vi "MM6.get i attribute.vi"(0 "i ref in":refnum<vi>, 5 "error in (no error)":errorcluster) -> (14 "i ref out":refnum<vi>, 16 "i attribute":T1={"ConfigData"={"GenConfig"={"Mode"=0, "Logs"=[]}, "Configs"=[]}, "UsedObjs"=[], "ActScanStep"=[], "AbortRequest"=FALSE, "StopRequest"=FALSE, "# cycles"=0, "Connected"=FALSE, "MMStatus"=enum."config", "# data"=0, "DIMServices"={"MM6StatusString"="", "MM6StatusID"=-1, "discArchiver"="", "discArchiverID"=-1, "eventBuilder"="", "eventBuilderID"=-1, "GUIIDString"="", "GUIIDStringID"=-1}, "dataFile"="", "ExtraDataSets"=[], "PGRunning"=0} {"ConfigData"."Configs"."CleanDev"."CleanData"."Time" format="%.3f"; "ConfigData"."Configs"."CleanDev"."CleanData"."Minus" format="%.2f"; "ConfigData"."Configs"."CleanDev"."CleanData"."Plus" format="%.2f"; "ConfigData"."Configs"."CleanDev"."CleanData"."Center" format="%.4f"; "ConfigData"."Configs"."CleanDev"."CleanData"."Amp" format="%.2f"; "ConfigData"."Configs"."Delays"."Delay" format="%.2f"; "ConfigData"."Configs"."Specials"."Data" format="%.2f"; "ConfigData"."Configs"."FreqDevs"."Time" format="%.3f"; "ConfigData"."Configs"."FreqDevs"."CenterFreq" format="%.4f"; "ConfigData"."Configs"."FreqDevs"."Amp" format="%.2f"; "ConfigData"."Configs"."Scans"."Values" format="%.2f"}, 19 "error out":errorcluster)   [LabVIEW 2014, in "MM6.lvlib"]
doc: "Gets the i attribute data of an object.\n\nLicense Agreement for this software:\n\nCopyright (C)\nGesellschaft für Schwerionenforschung, GSI\nPlanckstr. 1\n64291 Darmstadt\nGermany\n\nContact: D.Beck@gsi.de \n\nThis program is free software; you can redistribute it and/or modify it under the terms of the GNU General Public License as published by the Free Software Foundation; either version 2 of the license, or (at your option) any later version.\n\nThis program is distributed in the hope that it will be useful, but WITHOUT ANY WARRANTY; without even the implied warranty of MERCHANTABILITY or FITNESS FOR A PARTICULAR PURPOSE. See the GNU General License for more details (http://www.gnu.org).\n\nGesellschaft für Schwerionenforschung, GSI\nPlanckstr. 1, 64291 Darmstadt, Germany\nFor all questions and ideas contact: M.Richter@gsi.de, H.Brand@gsi.de or D.Beck@gsi.de.\nLast update: 17-JUN-2004"
uses:
  MM6.lvlib
  MM6.i attribute.ctl
  LEBITDefs/LEBITDefs.ConfigData.ctl
  LEBITDefs/LEBITDefs.GenConfig.ctl
  LEBITDefs/LEBITDefs.Log.ctl
  LEBITDefs/LEBITDefs.OneConfig.ctl
  LEBITDefs/LEBITDefs.MCA.ctl
  LEBITDefs/LEBITDefs.Timing.ctl
  LEBITDefs/LEBITDefs.Timetable.ctl
  LEBITDefs/LEBITDefs.Memory.ctl
  LEBITDefs/LEBITDefs.ScanDev.ctl
  LEBITDefs/LEBITDefs.FreqDev.ctl
  LEBITDefs/LEBITDefs.CleanDev.ctl
  LEBITDefs/LEBITDefs.CleanDataType.ctl
  LEBITDefs/LEBITDefs.Special.ctl
  LEBITDefs/LEBITDefs.Delay.ctl
  LEBITDefs/LEBITDefs.DAC.ctl
  MM6.status.ctl
  LEBITDefs/LEBITDefs.ExtraData.ctl
  CS_DigitalIO/PPG_ABC/PPG_ABC.PG_Running.ctl
  LEBITDefs/LEBITDefs.lvlib
  CS_DigitalIO/PPG_ABC/PPG_ABC.lvlib
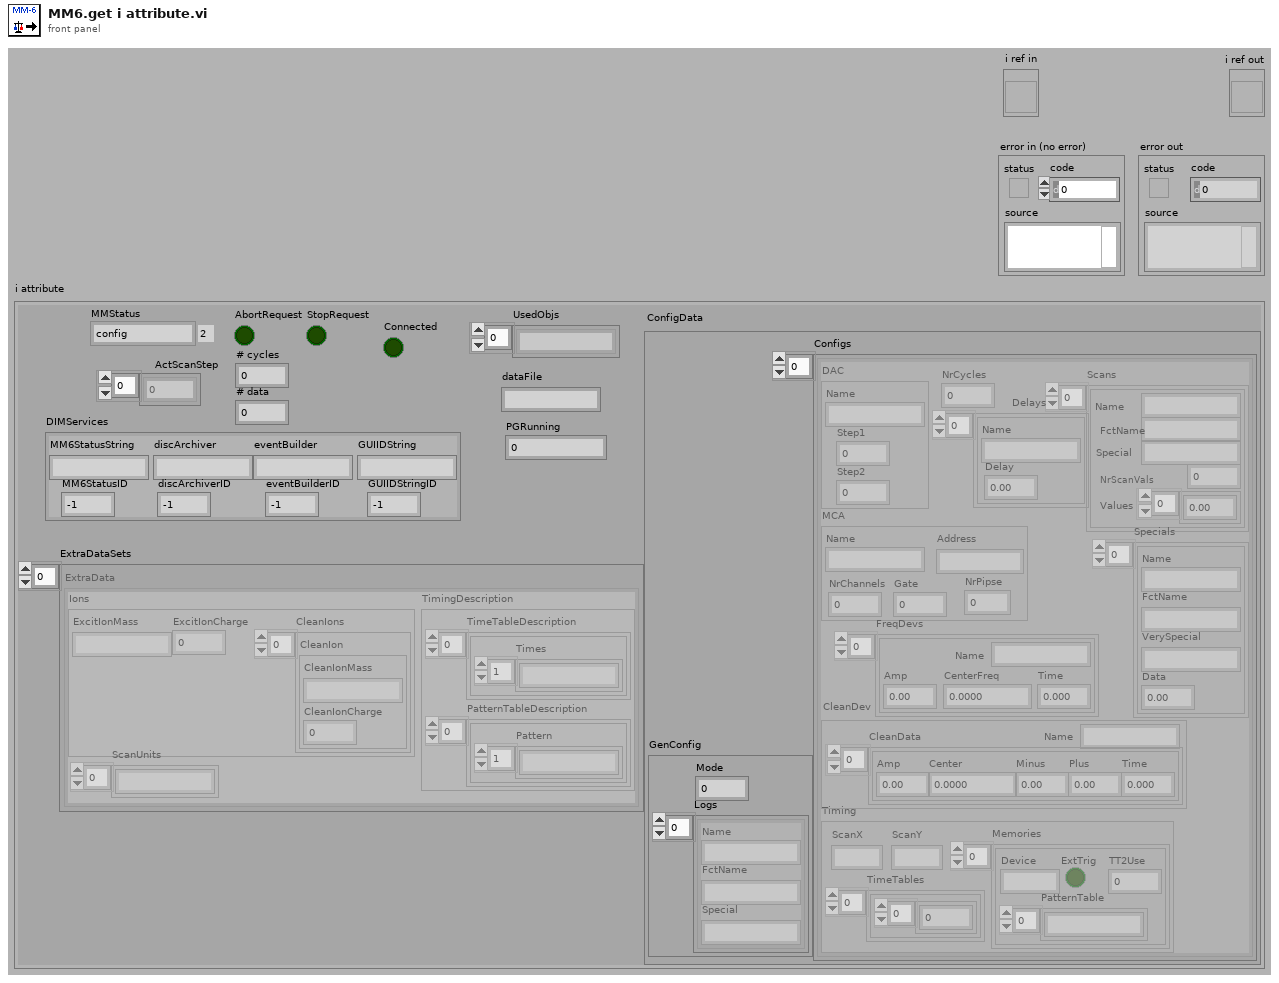
[diagram p1: front panel]
types:
  T1 = typedef "MM6.lvlib/MM6.i attribute.ctl" = cluster{"ConfigData":T2, "UsedObjs":string[], "ActScanStep":i32[], "AbortRequest":bool, "StopRequest":bool, "# cycles":i32, "Connected":bool, "MMStatus":T17, "# data":i32, "DIMServices":cluster{"MM6StatusString":string, "MM6StatusID":i32, "discArchiver":string, "discArchiverID":i32, "eventBuilder":string, "eventBuilderID":i32, "GUIIDString":string, "GUIIDStringID":i32}, "dataFile":string, "ExtraDataSets":T18, "PGRunning":T19}
  T2 = typedef "LEBITDefs.lvlib/LEBITDefs.ConfigData.ctl" = cluster{"GenConfig":T3, "Configs":T5[]}
  T3 = typedef "LEBITDefs.lvlib/LEBITDefs.GenConfig.ctl" = cluster{"Mode":i32, "Logs":T4[]}
  T4 = typedef "LEBITDefs.lvlib/LEBITDefs.Log.ctl" = cluster{"Name":string, "FctName":string, "Special":string}
  T5 = typedef "LEBITDefs.lvlib/LEBITDefs.OneConfig.ctl" = cluster{"MCA":T6, "Timing":T7, "Scans":T10[], "FreqDevs":T11[], "CleanDev":T12, "NrCycles":i32, "Specials":T14[], "Delays":T15[], "DAC":T16}
  T6 = typedef "LEBITDefs.lvlib/LEBITDefs.MCA.ctl" = cluster{"Name":string, "Address":string, "NrChannels":i32, "Gate":i32, "NrPipse":i32}
  T7 = typedef "LEBITDefs.lvlib/LEBITDefs.Timing.ctl" = cluster{"TimeTables":cluster{"TimeTable":T8}[], "Memories":T9[], "ScanX":string, "ScanY":string}
  T8 = typedef "LEBITDefs.lvlib/LEBITDefs.Timetable.ctl" = dbl[]
  T9 = typedef "LEBITDefs.lvlib/LEBITDefs.Memory.ctl" = cluster{"Device":string, "ExtTrig":bool, "TT2Use":i32, "PatternTable":string[]}
  T10 = typedef "LEBITDefs.lvlib/LEBITDefs.ScanDev.ctl" = cluster{"Name":string, "FctName":string, "Values":dbl[], "NrScanVals":i32, "Special":string}
  T11 = typedef "LEBITDefs.lvlib/LEBITDefs.FreqDev.ctl" = cluster{"Name":string, "Amp":dbl, "CenterFreq":dbl, "Time":dbl}
  T12 = typedef "LEBITDefs.lvlib/LEBITDefs.CleanDev.ctl" = cluster{"Name":string, "CleanData":T13[]}
  T13 = typedef "LEBITDefs.lvlib/LEBITDefs.CleanDataType.ctl" = cluster{"Amp":dbl, "Center":dbl, "Plus":dbl, "Minus":dbl, "Time":dbl}
  T14 = typedef "LEBITDefs.lvlib/LEBITDefs.Special.ctl" = cluster{"Name":string, "FctName":string, "VerySpecial":string, "Data":dbl}
  T15 = typedef "LEBITDefs.lvlib/LEBITDefs.Delay.ctl" = cluster{"Name":string, "Delay":dbl}
  T16 = typedef "LEBITDefs.lvlib/LEBITDefs.DAC.ctl" = cluster{"Name":string, "Step1":i32, "Step2":i32}
  T17 = typedef "MM6.lvlib/MM6.status.ctl" = enum16{"loaded", "load_error", "config", "config_error", "init", "init_error", "data_reset", "data_reset_error", "running", "start_error", "run_error", "abort_requested", "aborted", "stop_requested", "stopped", "stop_error", "Connected", "NOTConnected"}
  T18 = typedef "LEBITDefs.lvlib/LEBITDefs.ExtraData.ctl" = cluster{"Ions":cluster{"ExcitIonMass":string, "ExcitIonCharge":i32, "CleanIons":cluster{"CleanIonMass":string, "CleanIonCharge":i32}[]}, "TimingDescription":cluster{"TimeTableDescription":cluster{"Times":string[]}[], "PatternTableDescription":cluster{"Pattern":string[]}[]}, "ScanUnits":string[]}[]
  T19 = typedef "PPG_ABC.lvlib/PPG_ABC.PG_Running.ctl" = i32
  T20 = enum16{"SetAttribute", "GetAttribute", "CreateAttribute", "DestroyAttribute", "DestroyAllAtributes"}
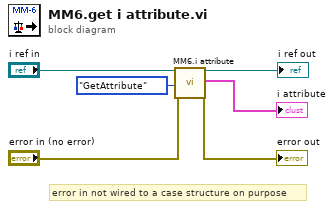
[diagram p0: block diagram]
diagram:
  # "error in not wired to a case structure on purpose"
  n1 = call "MM6.i attribute.vi"("VI Refnum"="i ref in", "Action"=T20."GetAttribute", "error in (no error)"="error in (no error)") -> ("VI Refnum out"=→"i ref out":refnum<vi>, "CLASS.i attribute out"=→"i attribute":T1, "error out"=→"error out":errorcluster)  [unwired: 14 in]
